vi "Update ATM Message.vi"(7 "Balance":dbl, 8 "error in (no error)":errorcluster, 9 "ATM Message Type":T1, 10 "Password":string, 11 "Path Account File":path) -> (0 "error out":errorcluster, 3 "ATM Messages":string)   [LabVIEW 2020]
doc: "This VI updates the ATM Message Indicator."
uses:
  Controls/ATM Message Types.ctl
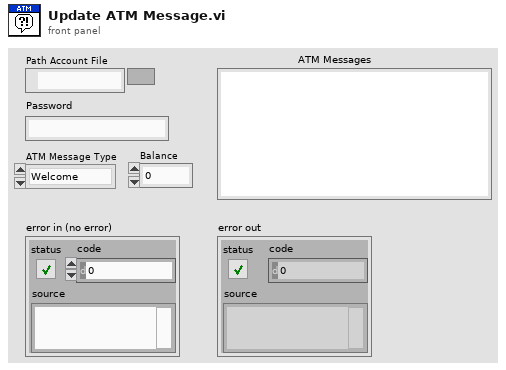
[diagram p1: front panel]
types:
  T1 = typedef "ATM Message Types.ctl" = enum16{"Welcome", "Main Menu", "Account Verification Failed", "Session Terminate Message", "Deposit ", "Deposit Completed", "Withdrawal", "Withdrawal Complete", "Withdrawal Failed", "Balance Inquiry"}
  T2 = cluster{"Balance":dbl, "Name":string, "Password":string}
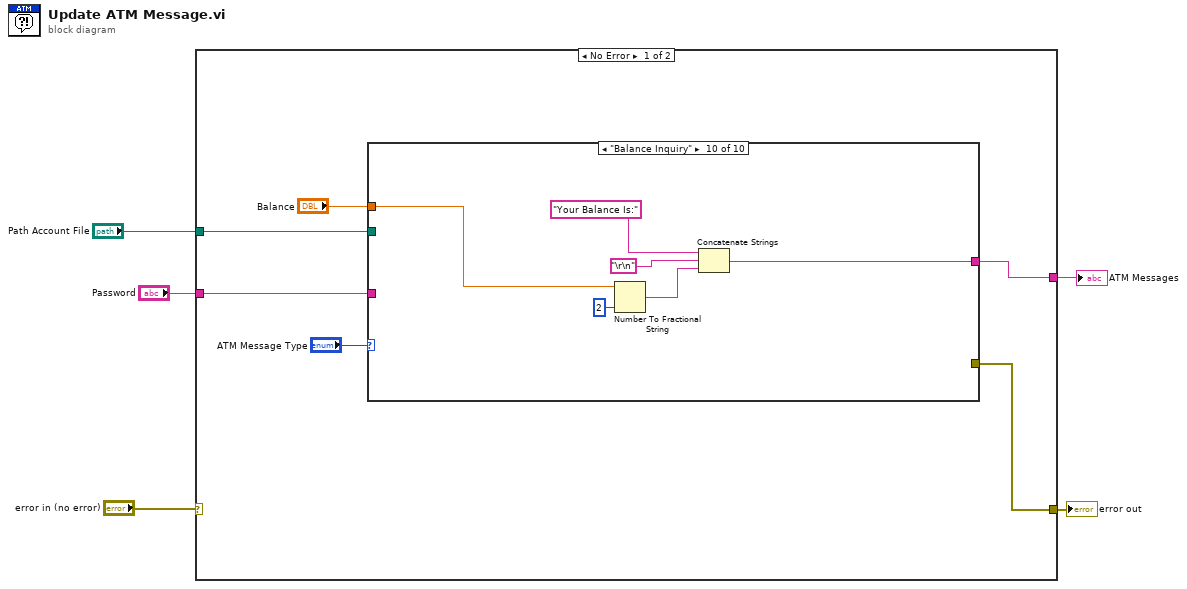
[diagram p0: block diagram]
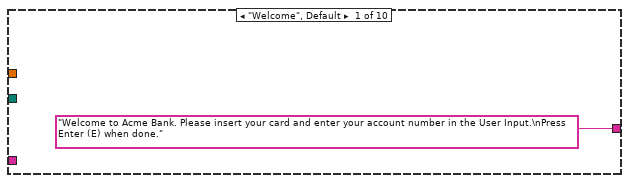
[diagram p2: hidden frame]
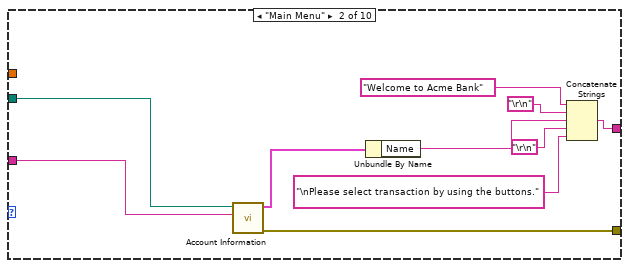
[diagram p3: hidden frame]
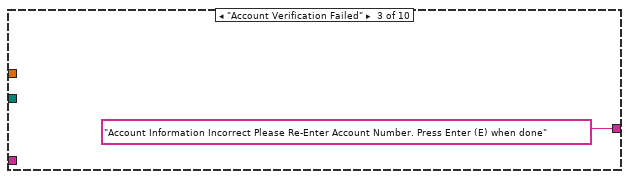
[diagram p4: hidden frame]
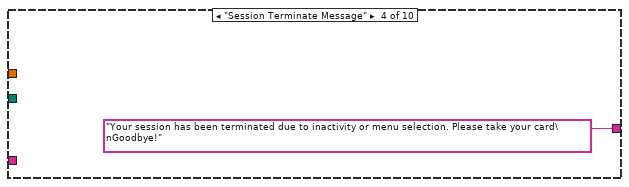
[diagram p5: hidden frame]
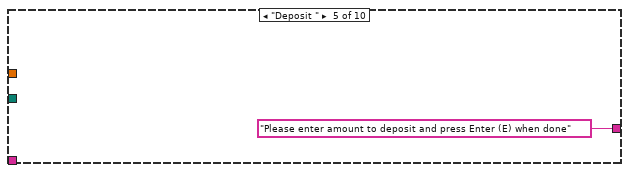
[diagram p6: hidden frame]
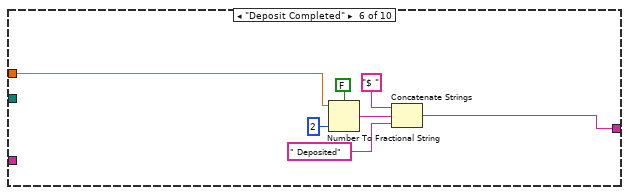
[diagram p7: hidden frame]
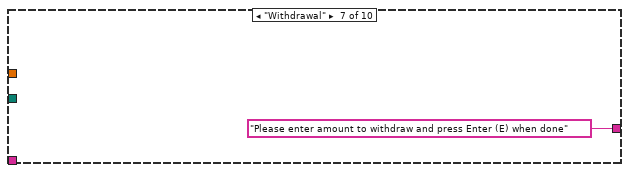
[diagram p8: hidden frame]
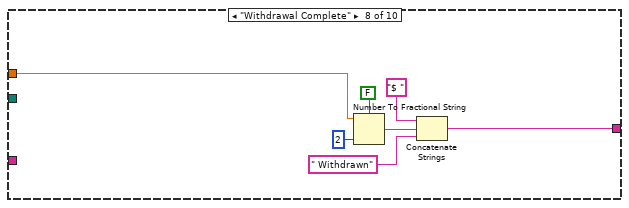
[diagram p9: hidden frame]
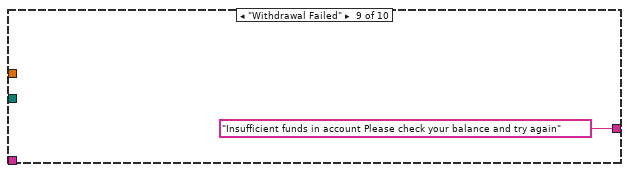
[diagram p10: hidden frame]
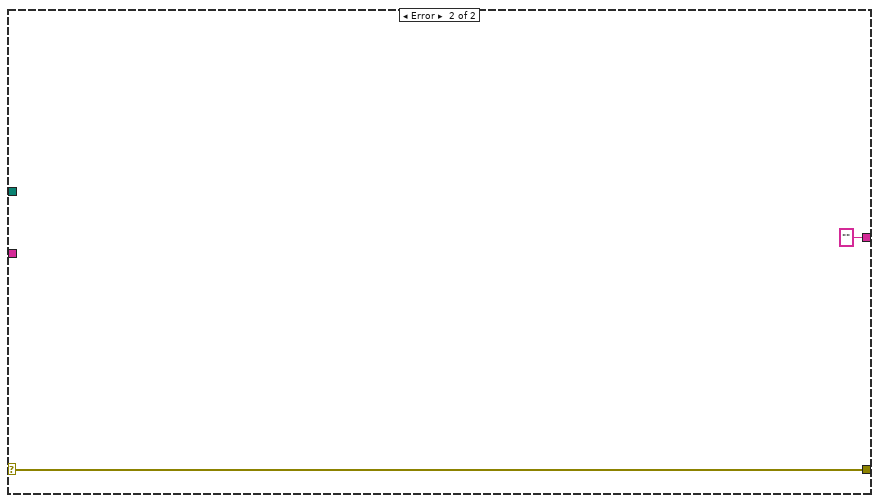
[diagram p11: hidden frame]
diagram:
  n1 = case shown="No Error" "error in (no error)" {
    selector: "error in (no error)" -> [_ w49]
    tunnel: [w8 w49] -> w2
    tunnel: [w10 "" ("ATM Messages")] -> w3
    tunnel: "Path Account File" -> [w9 _]
    tunnel: "Password" -> [w7 _]
    frame No Error {
      n2 = case shown="\"Balance Inquiry\"" "ATM Message Type" {
        tunnel: ["Welcome to Acme Bank. Please insert your card and enter your account number in the User Input.\nPress Enter (E) when done." ("ATM Messages") w17 "Account Information Incorrect Please Re-Enter Account Number. Press Enter (E) when done" ("ATM Messages") "Your session has been terminated due to inactivity or menu selection. Please take your card\nGoodbye!" ("ATM Messages") "Please enter amount to deposit and press Enter (E) when done" ("ATM Messages") w29 "Please enter amount to withdraw and press Enter (E) when done" ("ATM Messages") w37 "Insufficient funds in account Please check your balance and try again" ("ATM Messages") w42] -> w10
        tunnel: w9 -> [_ w21 _ _ _ _ _ _ _ _]
        tunnel: [_ w22 _ _ _ _ _ _ _ _] -> w8
        tunnel: w7 -> [_ w20 _ _ _ _ _ _ _ _]
        tunnel: "Balance" -> [_ _ _ _ _ w28 _ w36 _ w45]
        frame "Welcome", Default {
        }
        frame "Main Menu" {
          n3 = call "Account Information.vi"("Password"=w20, "file path (dialog if empty)"=w21) -> ("error out"=w22:errorcluster, "Account Information"=w19:T2)  [unwired: 8 in]
          n4 = Unbundle By Name(w19) -> ("Name"=w15:string)
          n5 = Concatenate Strings("Welcome to Acme Bank" ("ATM Messages"), "\r\n", w15, "\r\n", "\nPlease select transaction by using the buttons." ("string")) -> (w17:string)
        }
        frame "Account Verification Failed" {
        }
        frame "Session Terminate Message" {
        }
        frame "Deposit " {
        }
        frame "Deposit Completed" {
          n6 = Number To Fractional String(use system decimal point (T)=FALSE, number=w28, precision (6)=i16 2) -> (F-format string=w32:string)  [unwired: 1 in]
          n7 = Concatenate Strings("$ " ("string"), w32, " Deposited" ("string")) -> (w29:string)
        }
        frame "Withdrawal" {
        }
        frame "Withdrawal Complete" {
          n8 = Number To Fractional String(use system decimal point (T)=FALSE, number=w36, precision (6)=i16 2) -> (F-format string=w40:string)  [unwired: 1 in]
          n9 = Concatenate Strings("$ " ("string"), w40, " Withdrawn" ("string")) -> (w37:string)
        }
        frame "Withdrawal Failed" {
        }
        frame "Balance Inquiry" {
          n10 = Number To Fractional String(number=w45, precision (6)=i16 2) -> (F-format string=w43:string)  [unwired: 2 in]
          n11 = Concatenate Strings("Your Balance Is:" ("string"), "\r\n", w43) -> (w42:string)
        }
      }
    }
    frame Error {
    }
  }
  "error out" <- w2
  "ATM Messages" <- w3
